vi "Load SLSC Switch Module Configuration.vi"(6 "Model":string, 8 "error in":errorcluster, 9 "Resource":string, 10 "switches JSON file":path, 11 "SLSC Switch Custom Device Ref in":T1 format="%.0x") -> (0 "error out":errorcluster, 3 "SLSC Switch Custom Device Ref out":T1 format="%.0x")   [LabVIEW 2017, in "SLSC Switch Scripting.lvlib"]
uses:
  SLSC Switch Scripting.lvlib
  <vilib>/NI Veristand/Custom Device API/Custom Device Item Ref.ctl
  <vilib>/NI Veristand/Custom Device API/Custom Device API.lvlib
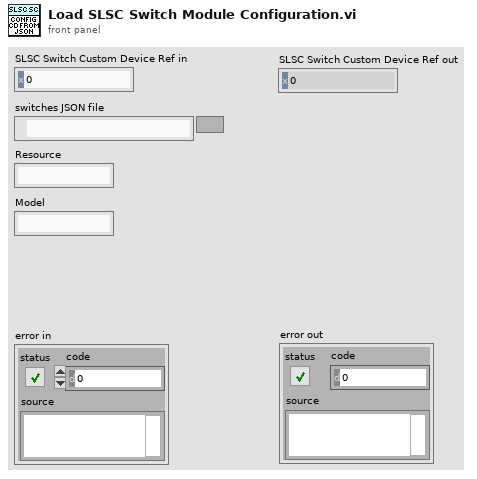
[diagram p1: front panel]
types:
  T1 = typedef "Custom Device API.lvlib/Custom Device Item Ref.ctl" = u64
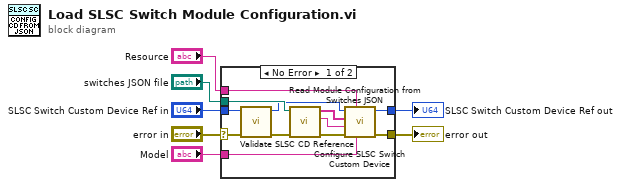
[diagram p0: block diagram]
diagram:
  n1 = case shown="No Error" "error in" {
    selector: "error in" -> [w9 w20]
    tunnel: "SLSC Switch Custom Device Ref in" -> [w11 w21]
    tunnel: [w17 w20] -> w4
    tunnel: [w18 w21] -> w5
    tunnel: "switches JSON file" -> [w16 _]
    tunnel: "Resource" -> [w14 _]
    tunnel: "Model" -> [w15 _]
    frame No Error {
      n2 = call "Validate SLSC CD Reference.vi"("error in (no error)"=w9, "SLSC Switch Custom Device Ref in"=w11) -> ("error out"=w8:errorcluster, "SLSC Switch Custom Device Ref out"=w10:T1)  [unwired: 8 in]
      n3 = call "Read Module Configuration from Switches JSON.vi"("error in (no error)"=w8, "switches JSON file"=w16) -> ("error out"=w19:errorcluster, "switches json"=w12:string, "topologies"=w13:string[])  [unwired: 7 in]
      n4 = call "Configure SLSC Switch Custom Device.vi"("model"=w15, "resource"=w14, "error in (no error)"=w19, "switches json"=w12, "topologies"=w13, "SLSC Switch Custom Device Ref in"=w10) -> ("error out"=w17:errorcluster, "SLSC Switch Custom Device Ref out"=w18:T1)  [unwired: 4 in]
    }
    frame Error {
    }
  }
  "error out" <- w4
  "SLSC Switch Custom Device Ref out" <- w5
